vi "To Pairs.vi"(4 "Elements":string[](array[string])) -> (1 "Array":string[][](array[string]))   [LabVIEW 2016, in "Horizontal MenuList.xctl"]
uses:
  Horizontal MenuList.xctl
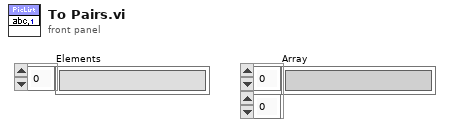
[diagram p1: front panel]
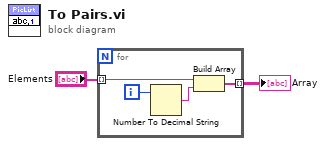
[diagram p0: block diagram]
diagram:
  n1 = for {
    tunnel: "Elements" -> [w5] mode=indexing
    tunnel: [w3] -> w1 mode=indexing
    i -> [w6]
    n2 = Number To Decimal String(number=w6) -> (decimal integer string=w4:string)  [unwired: 1 in]
    n3 = Build Array(w5, w4) -> (w3:string[])
  }
  "Array" <- w1
